vi "Add To Child List.vi"(10 "Child ID":string, 11 "Generic Node in":refnum<class "Generic Node.lvclass">) -> (3 "Generic Node out":refnum<class "Generic Node.lvclass">)   [LabVIEW 2017, in "opcua.lvlib" / "Browser Core.lvlib" / "Generic Node.lvclass"]
doc: "Add Child ID to parent's list of children"
uses:
  Generic Node.lvclass
  Generic Node.lvclass/Generic Node.ctl
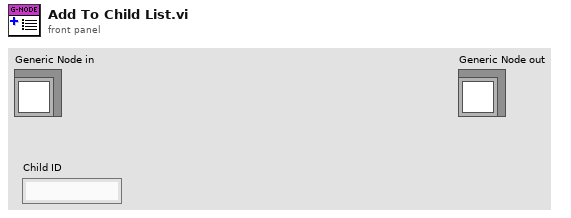
[diagram p1: front panel]
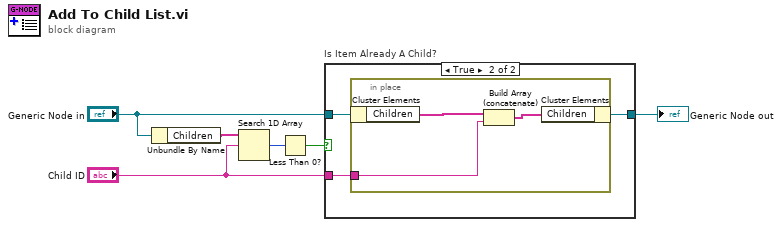
[diagram p0: block diagram]
diagram:
  n1 = Unbundle By Name("Generic Node in") -> ("Children"=w4:string[])
  n2 = Search 1D Array(1D array=w4, element="Child ID") -> (index of element=w3:i32)  [unwired: 1 in]
  n3 = Less Than 0?(x=w3) -> (x < 0?=w2:bool)
  n4 = case "Is Item Already A Child?" shown="True" w2 {
    tunnel: [w7 w8] -> w6
    tunnel: "Generic Node in" -> [w7 w10]
    tunnel: "Child ID" -> [_ w9]
    frame False {
    }
    frame True {
      n5 = in-place {
        in-place-border: w9 -> [w12]
        n6 = in-place-cluster #1(w10) -> ("Children"=w13:string[])
        n7 = Build Array (concatenate)(w13, w12) -> (w11:string[])
        n8 = in-place-cluster #1("Children"=w11) -> (w8:refnum<class "Generic Node.lvclass">)
      }
    }
  }
  "Generic Node out" <- w6
